vi "cascade_control_example.vi"() -> ()   [LabVIEW 2015]
doc: "This example shows you a classical feedback control loop with a PID controller and a simulated process that behaves as a second order transfer function. You can ignore the settings for the simulated process if you want and focus on tunning the controller. You can also change the parameters of the simulated process in order to make them behave differently (i.e. oscillate more, have less overshoot, etc)."
uses:
  discrete_control_systems/discrete_control_systems.lvlib
panel:
  in  "Outer Manual Input":dbl
  in  "Closed Loop?":enum32{"Closed Loop", "Open Loop"}(radio)
  in  "Closed Loop?":enum32{"Closed Loop", "Open Loop"}(radio)
  out "Inner PV":dbl=4.499787600733511
  in  "Inner SP":dbl
  in  "PID Parameters":cluster{"Kc":dbl, "Ti":dbl, "Td":dbl}={"Kc"=0.08, "Ti"=0.07, "Td"=0.25}
  in  "PID Output Limits":cluster{"Max":dbl, "Min":dbl}={"Max"=10.0, "Min"=-10.0}
  in  "Reset Controller":bool
  in  "Reset Plant":bool
  in  "Simulation Output Limits":cluster{"Max":dbl, "Min":dbl}={"Max"=200.0, "Min"=-200.0}
  in  "Simulation Parameters":T1={"Gain"=2.0, "NaturalFreq (wn in Hz)"=1.0, "DampingRatio (zeta)"=0.3} caption="Outer Simulated Process"
  in  "Simulation Parameters":T1={"Gain"=2.0, "NaturalFreq (wn in Hz)"=7.0, "DampingRatio (zeta)"=0.2} caption="Inner Simulated Process"
  in  "PID Parameters":cluster{"Kc":dbl, "Ti":dbl, "Td":dbl}={"Kc"=0.07, "Ti"=0.005, "Td"=0.1}
  in  "Sampling Time(s)":dbl=0.01 format="%#_13g"
  in  "Closed Loop?":enum32{"Closed Loop", "Open Loop"}(radio)
  in  "Inner Manual Input":dbl
  out "Process Chart":T2(graph)={"Set Point"=9.0, "Manual Input (Open Loop)"=2.249897039132027, "output"=4.499787600733511, "output"=8.999147687970632}
  in  "Stop":bool
  out "Process Variable":dbl=8.999147687970632
  in  "Reset Plant":bool
  in  "Simulation Output Limits":cluster{"Max":dbl, "Min":dbl}={"Max"=200.0, "Min"=-200.0}
  out "Control Value":dbl=2.249897039132027
  in  "Set Point":dbl
  in  "PID Output Limits":cluster{"Max":dbl, "Min":dbl}={"Max"=10.0, "Min"=-10.0}
  in  "Reset Controller":bool
  # "JKI DISCRETE CONTROL SYSTEMS\nCascade closed loop control example\nThis example shows how to implement a cascade control stragery with 2 PIDs and 2 processes. Typically, for a cascade strategy to work, the inner process has to respond faster than the outer process. A classic example is the \nlevel control of a tank with an electronic valve as the actuator. In that case, the electronic valve would be the inner\nprocess that you want to control and make it go to a desired position. The outer process would be the level of the tank."
  # "INNER PROCESS"
  # "OUTER PROCESS"
  # "INNER PID"
  # "OUTER PID"
  # "You can change the setpoint\nwhen running closed loop"
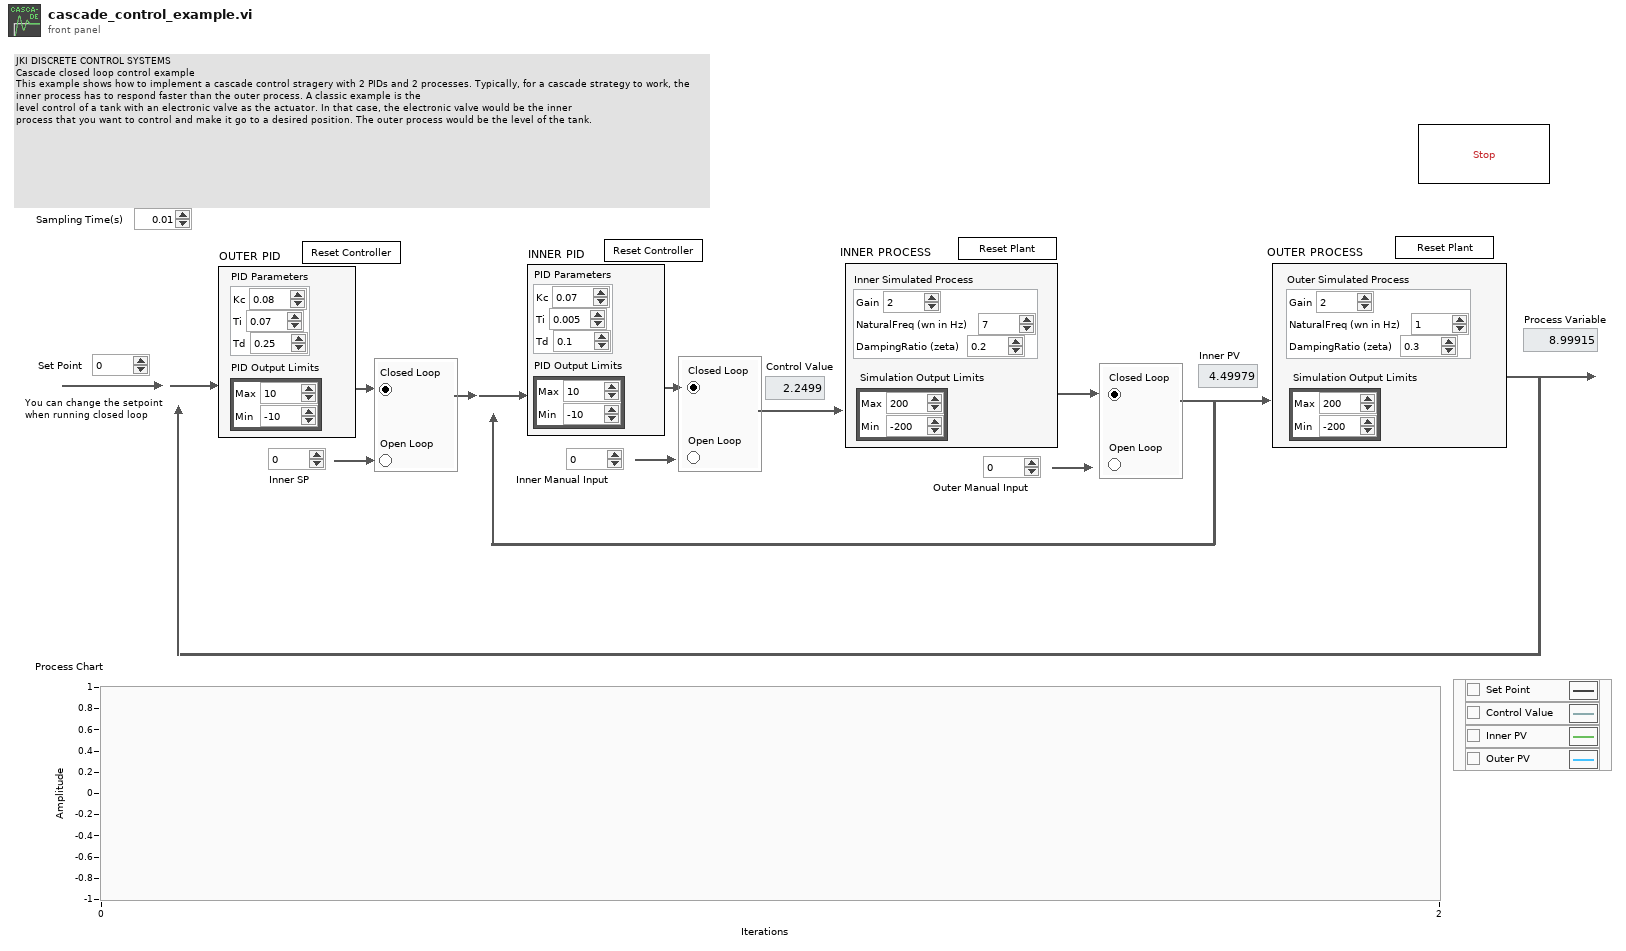
[diagram p1: front panel]
types:
  T1 = cluster{"Gain":dbl, "NaturalFreq (wn in Hz)":dbl, "DampingRatio (zeta)":dbl}
  T2 = cluster{"Set Point":dbl, "Manual Input (Open Loop)":dbl, "output":dbl, "output":dbl}
  T3 = cluster{"Set Point":dbl, "Inner Manual Input":dbl, "output":dbl, "output":dbl}
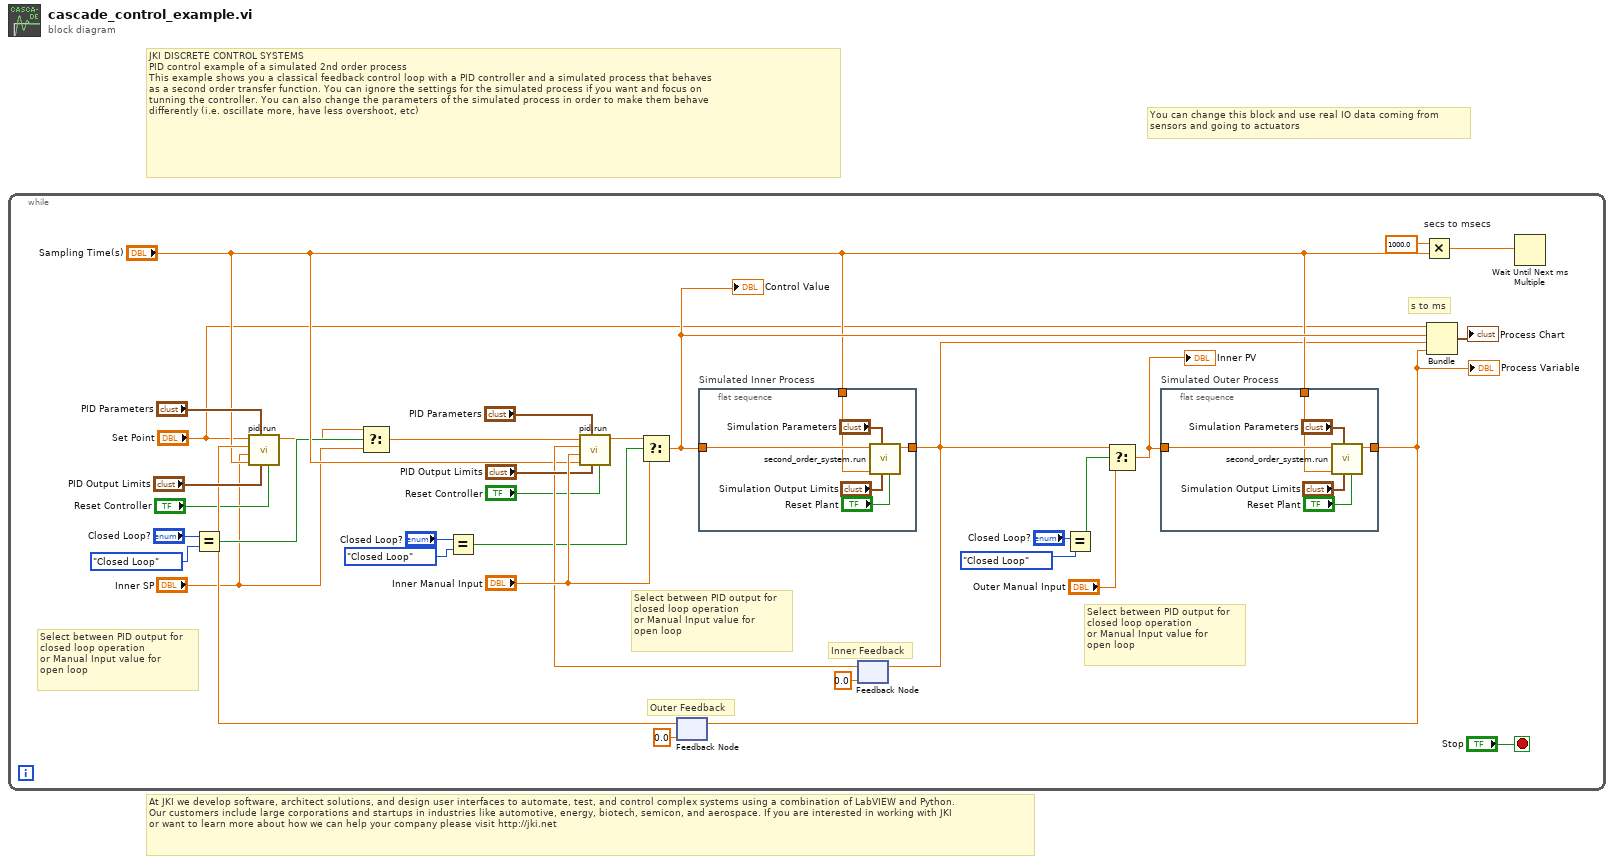
[diagram p0: block diagram]
diagram:
  # "You can change this block and use real IO data coming from\nsensors and going to actuators"
  # "JKI DISCRETE CONTROL SYSTEMS\nPID control example of a simulated 2nd order process\nThis example shows you a classical feedback control loop with a PID controller and a simulated process that behaves \nas a second order transfer function. You can ignore the settings for the simulated process if you want and focus on\ntunning the controller. You can also change the parameters of the simulated process in order to make them behave\ndifferently (i.e. oscillate more, have less overshoot, etc)"
  # "At JKI we develop software, architect solutions, and design user interfaces to automate, test, and control complex systems using a combination of LabVIEW and Python. \nOur customers include large corporations and startups in industries like automotive, energy, biotech, semicon, and aerospace. If you are interested in working with JKI\nor want to learn more about how we can help your company please visit http://jki.net"
  n1 = while {
    stop <- "Stop" stop-if-true
    # "Select between PID output for\nclosed loop operation\nor Manual Input value for \nopen loop"
    # "Select between PID output for\nclosed loop operation\nor Manual Input value for \nopen loop"
    # "Outer Feedback"
    # "Select between PID output for\nclosed loop operation\nor Manual Input value for \nopen loop"
    # "s to ms"
    # "Inner Feedback"
    n2 = Equal?(x="Closed Loop?", y=enum32{"Closed Loop", "Open Loop"}."Closed Loop") -> (x = y?=w11:bool)
    n3 = Equal?(x="Closed Loop?", y=enum32{"Closed Loop", "Open Loop"}."Closed Loop") -> (x = y?=w22:bool)
    n4 = feedback #1(0.0 ("y(k)")) -> (w17:dbl)
    n5 = call "pid.run.vi"("reset? (F)"="Reset Controller", "output_limits (100/0)"="PID Output Limits", "pid_parameters"="PID Parameters", "sampling_time (s)"="Sampling Time(s)", "initial_output (0)"="Inner SP", "feedback"=w17, "setpoint"="Set Point") -> ("controller_output"=w10:dbl)  [unwired: 4 in]
    n6 = Select(t=w10, s=w11, f="Inner SP") -> (s? t:f=w9:dbl)
    n7 = feedback-in #1(w18) -> ()
    n8 = flat-sequence "Simulated Inner Process" {
      tunnel: w24 -> [w45]
      tunnel: [w44] -> w6
      tunnel: "Sampling Time(s)" -> [w42]
      frame #0 {
        n9 = call "second_order_system.run.vi"("reset? (F)"="Reset Plant", "output_limits (100/0)"="Simulation Output Limits", "transfer_function_parameters"="Simulation Parameters", "sampling_time (s)"=w42, "input"=w45) -> ("output"=w44:dbl)  [unwired: 6 in]
      }
    }
    n10 = feedback-in #2(w6) -> ()
    n11 = feedback #2(0.0 ("y(k)")) -> (w23:dbl)
    n12 = call "pid.run.vi"("reset? (F)"="Reset Controller", "output_limits (100/0)"="PID Output Limits", "pid_parameters"="PID Parameters", "sampling_time (s)"="Sampling Time(s)", "initial_output (0)"="Inner Manual Input", "feedback"=w23, "setpoint"=w9) -> ("controller_output"=w25:dbl)  [unwired: 4 in]
    n13 = Select(t=w25, s=w22, f="Inner Manual Input") -> (s? t:f=w24:dbl)
    "Control Value" <- w24
    n14 = Equal?(x="Closed Loop?", y=enum32{"Closed Loop", "Open Loop"}."Closed Loop") -> (x = y?=w4:bool)
    n15 = Select(t=w6, s=w4, f="Outer Manual Input") -> (s? t:f=w5:dbl)
    "Inner PV" <- w5
    n16 = flat-sequence "Simulated Outer Process" {
      tunnel: w5 -> [w39]
      tunnel: [w38] -> w18
      tunnel: "Sampling Time(s)" -> [w36]
      frame #0 {
        n17 = call "second_order_system.run.vi"("reset? (F)"="Reset Plant", "output_limits (100/0)"="Simulation Output Limits", "transfer_function_parameters"="Simulation Parameters", "sampling_time (s)"=w36, "input"=w39) -> ("output"=w38:dbl)  [unwired: 6 in]
      }
    }
    n18 = Multiply "secs to msecs"(x=1000.0, y="Sampling Time(s)") -> (x*y=w29:dbl)
    n19 = Bundle("Set Point"="Set Point", "Inner Manual Input"=w24, "output"=w6, "output"=w18) -> (→"Process Chart":T3)  [unwired: 1 in]
    n20 = Wait Until Next ms Multiple(millisecond multiple=w29) -> ()  [unwired: 1 out]
    "Process Variable" <- w18
  }
